vi "BuildSlaveRWr.vi"() -> (0 "RWr":i16[][](array[numeric]))   [LabVIEW 2018]
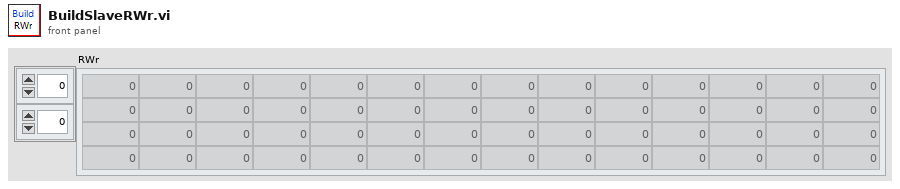
[diagram p1: front panel]
types:
  T1 = cluster{"轮盘预压力":sgl, "泄漏量上限":sgl, "压力上限":sgl, "压力下限":sgl, "风门闭电压上限":sgl, "风门闭电压下限":sgl, "风门开电压上限":sgl, "风门开电压下限":sgl, "LED电流上限":sgl, "LED电流下限":sgl, "气压稳定时间":sgl, "伺服速度":sgl}
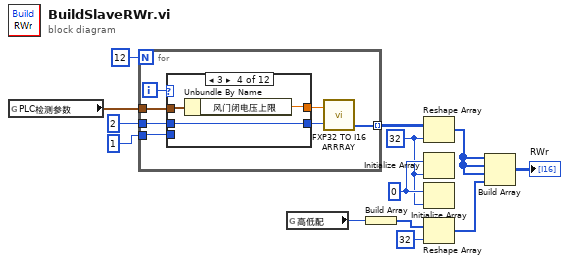
[diagram p0: block diagram]
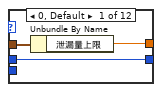
[diagram p2: hidden frame]
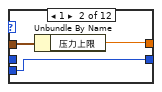
[diagram p3: hidden frame]
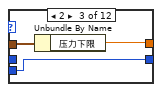
[diagram p4: hidden frame]
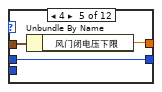
[diagram p5: hidden frame]
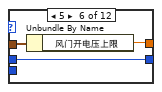
[diagram p6: hidden frame]
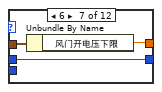
[diagram p7: hidden frame]
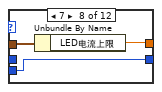
[diagram p8: hidden frame]
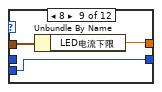
[diagram p9: hidden frame]
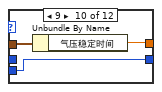
[diagram p10: hidden frame]
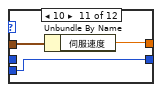
[diagram p11: hidden frame]
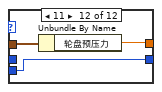
[diagram p12: hidden frame]
diagram:
  w8 = i16 0
  w7 = 32 ("维数大小")
  n1 = global read "全局 1.vi" "PLC检测参数"() -> (w13:T1)
  n2 = for {
    N: 12 -> [_]
    tunnel: w13 -> [w20]
    tunnel: 2 ("位数(2)") -> [w19]
    tunnel: [w15] -> w9 mode=indexing
    tunnel: 1 ("位数(2)") -> [w14]
    i -> [w18]
    n3 = case shown="3" w18 {
      tunnel: w20 -> [w23 w26 w29 w32 w35 w38 w41 w44 w47 w50 w53 w56]
      tunnel: w19 -> [w21 _ _ w30 w33 w36 w39 _ _ _ _ _]
      tunnel: [w22 w25 w28 w31 w34 w37 w40 w43 w46 w49 w52 w55] -> w17
      tunnel: [w21 w24 w27 w30 w33 w36 w39 w42 w45 w48 w51 w54] -> w16
      tunnel: w14 -> [_ w24 w27 _ _ _ _ w42 w45 w48 w51 w54]
      frame 0, Default {
        n4 = Unbundle By Name(w23) -> ("泄漏量上限"=w22:sgl)
      }
      frame 1 {
        n5 = Unbundle By Name(w26) -> ("压力上限"=w25:sgl)
      }
      frame 2 {
        n6 = Unbundle By Name(w29) -> ("压力下限"=w28:sgl)
      }
      frame 3 {
        n7 = Unbundle By Name(w32) -> ("风门闭电压上限"=w31:sgl)
      }
      frame 4 {
        n8 = Unbundle By Name(w35) -> ("风门闭电压下限"=w34:sgl)
      }
      frame 5 {
        n9 = Unbundle By Name(w38) -> ("风门开电压上限"=w37:sgl)
      }
      frame 6 {
        n10 = Unbundle By Name(w41) -> ("风门开电压下限"=w40:sgl)
      }
      frame 7 {
        n11 = Unbundle By Name(w44) -> ("LED电流上限"=w43:sgl)
      }
      frame 8 {
        n12 = Unbundle By Name(w47) -> ("LED电流下限"=w46:sgl)
      }
      frame 9 {
        n13 = Unbundle By Name(w50) -> ("气压稳定时间"=w49:sgl)
      }
      frame 10 {
        n14 = Unbundle By Name(w53) -> ("伺服速度"=w52:sgl)
      }
      frame 11 {
        n15 = Unbundle By Name(w56) -> ("轮盘预压力"=w55:sgl)
      }
    }
    n16 = call "FXP32 TO I16 ARRRAY.vi"("FXP32in"=w17, "位数(2)"=w16) -> ("out I16 array"=w15:i16[])  [unwired: 2 out]
  }
  n17 = global read "全局 1.vi" "高低配"() -> (w6:i16)
  n18 = Build Array(w6) -> (w5:i16[])
  n19 = Reshape Array ("重排数组维数")(w9, w7) -> (w1:i16[])
  n20 = Initialize Array(w8, w7) -> ()  [unwired: 1 out]
  n21 = Initialize Array(w8, w7) -> ()  [unwired: 1 out]
  n22 = Reshape Array(w5, 32 ("维数大小")) -> (w3:i16[])
  n23 = Build Array(w1, w1, w1, w3) -> (→"RWr":i16[][])
